vi "3. CoffeeMaker Initialize and Stop.vi"() -> ()   [LabVIEW 2018]
doc: "Coffee Machine Version 1.0: initializing and stopping the state machine"
uses:
  Controls/States.ctl
panel:
  out "error out":errorcluster
  in  "error in (no error)":errorcluster
  in  "Power Switch":bool
  in  "Simulation":cluster{"Water":dbl, "Coffee":dbl, "Milk":dbl} {"Milk" scale=0.0..100.0; "Water" scale=0.0..100.0; "Coffee" scale=0.0..100.0}
  out "Display":T1 {"Coffee" scale=0.0..80.0; "Brewing Chamber" scale=0.0..80.0}
  in  "Control \nElements":T2 {"Type" min=0 max=2 scale=0.0..2.0}
  # "Coffee Selection"
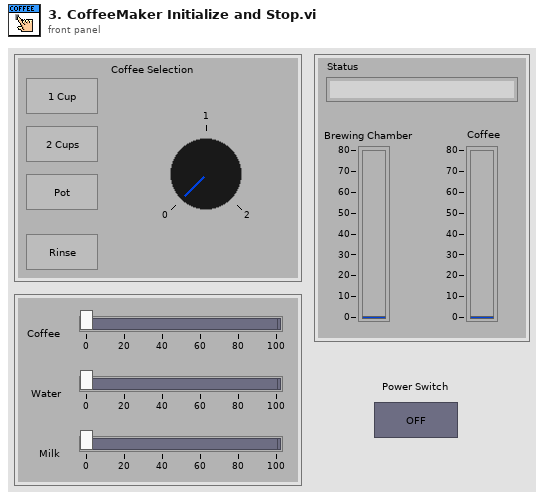
[diagram p1: front panel]
types:
  T1 = cluster{"Brewing Chamber":dbl, "Coffee":dbl, "Status":string}
  T2 = cluster{"1 Cup":bool, "2 Cups":bool, "Pot":bool, "Rinse":bool, "Type":i8}
  T3 = typedef "States.ctl" = enum16{"Initialize", "Set Language", "Wait for Power On", "Heat up", "Check and Wait for Water", "Rinsing", "Check Resources", "User Input", "Grinding", "Boiling", "Pouring", "Rinse before Stop", "Write Data", "Stop"}
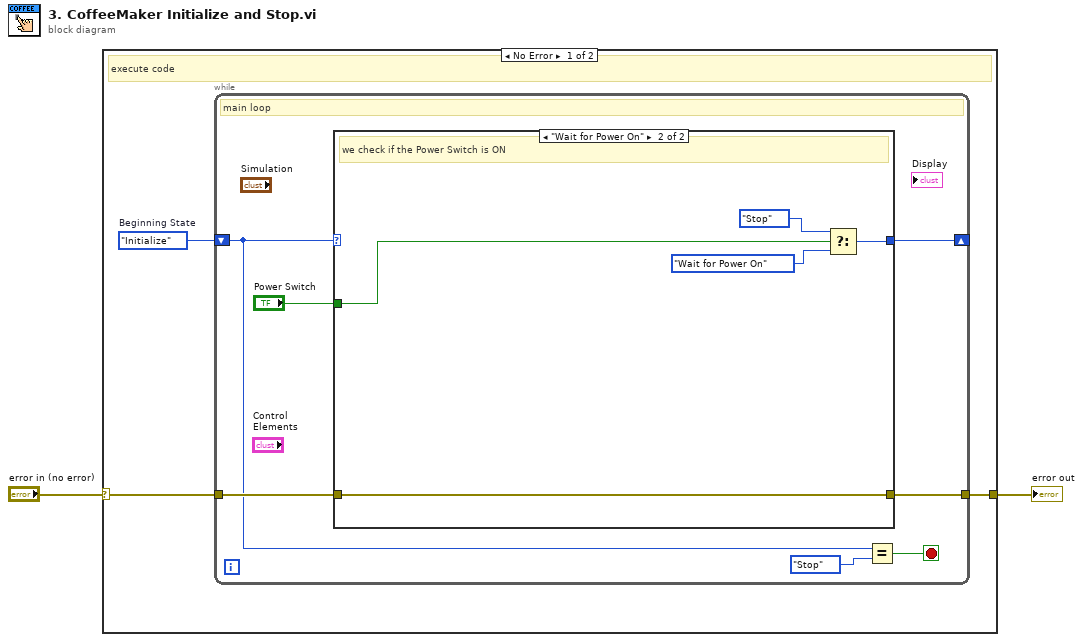
[diagram p0: block diagram]
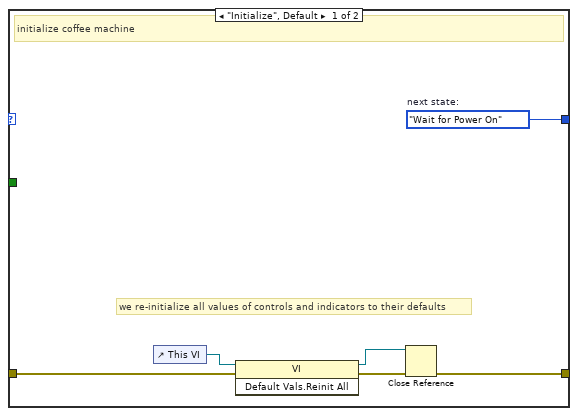
[diagram p2: hidden frame]
diagram:
  n1 = case shown="No Error" "error in (no error)" {
    selector: "error in (no error)" -> [w4 w24]
    tunnel: [w5 w24] -> w1
    frame No Error {
      w3 = States."Initialize"  # Beginning State
      # "execute code"
      n2 = while {
        tunnel: [w12] -> w5
        tunnel: w4 -> [w11]
        shift-right: [w9] -> _
        shift-left: w3 -> [w8]
        stop <- w6 stop-if-true
        # "main loop"
        n3 = case shown="\"Wait for Power On\"" w8 {
          tunnel: [w14 w19] -> w12
          tunnel: w11 -> [w17 w19]
          tunnel: "Power Switch" -> [_ w23]
          tunnel: [w13 w22] -> w9
          frame "Initialize", Default {
            w13 = States."Wait for Power On"  # next state:
            # "we re-initialize all values of controls and indicators to their defaults"
            # "initialize coffee machine"
            n4 = control-ref of="This VI"() -> (w18:refnum<vi>)
            n5 = invoke class="VI" method="Default Vals.Reinit All"(reference=w18, error in=w17) -> (reference out=w16:refnum<vi>, error out=w15:errorcluster)  [unwired: 1 in, 1 out]
            n6 = Close Reference(reference=w16, error in (no error)=w15) -> (error out=w14:errorcluster)
          }
          frame "Wait for Power On" {
            # "we check if the Power Switch is ON"
            n7 = Select(t=States."Stop" ("Beginning State"), s=w23, f=States."Wait for Power On") -> (s? t:f=w22:T3)
          }
        }
        n8 = Equal?(x=w8, y=States."Stop") -> (x = y?=w6:bool)
      }
    }
    frame Error {
      # "do nothing"
    }
  }
  "error out" <- w1
